vi "ASCENSOR.vi"() -> ()   [LabVIEW 2019]
panel:
  in  "Bajar":bool
  in  "Subir":bool
  in  "Posicion Ascensor":dbl(slide) scale=0.0..100.0
  in  "Selecc. Piso Inicio":enum16{"Piso 1", "Piso 2", "Piso 3", "Piso 4"}(ring)
  in  "Manual-Automatico":bool=TRUE
  in  "Start-Stop":bool
  in  "Cerrar":bool
  in  "Abrir":bool
  out "Bajando":bool
  out "Subiendo":bool
  in  "Piso 4":u16(ring)
  in  "Piso 3":u16(ring)
  in  "Piso 2":u16(ring)
  in  "Piso 1":u16(ring)
  in  "Indicador Cabina":u16(ring)
  out "Bajar 4":bool
  out "Subir 3":bool
  out "Bajar 3":bool
  out "Subir 2":bool
  out "Bajar 2":bool
  out "Subir 1":bool
  out "P02":bool
  out "P04":bool
  out "P01":bool
  out "P03":bool
  in  "Piso 4":bool
  in  "Piso 2":bool
  in  "Piso 3":bool
  in  "Piso 1":bool
  # "0 = Piso 1"
  # "33 = Piso 2"
  # "66 = Piso 3"
  # "100 = Piso 4"
  # "Operacion Manual"
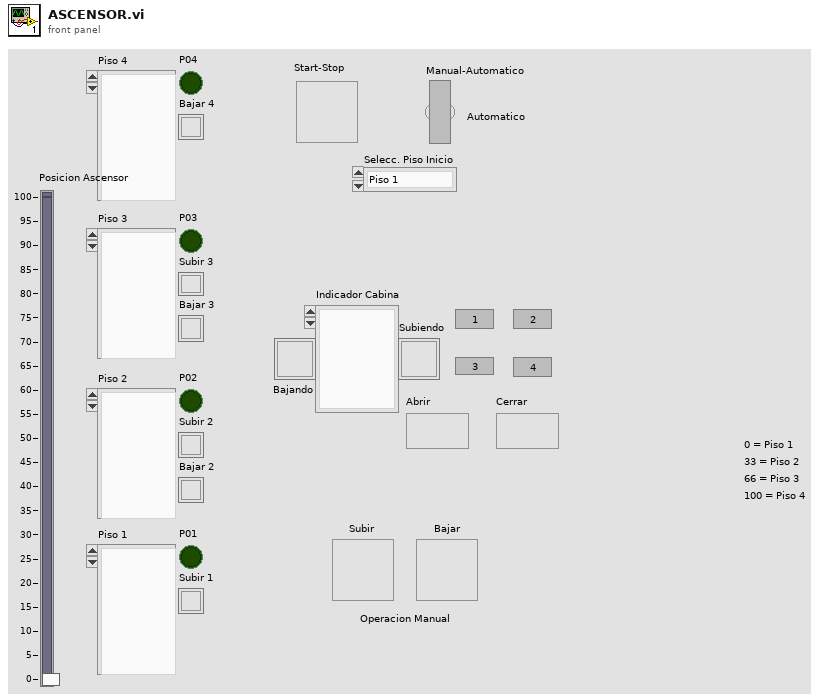
[diagram p1: front panel]
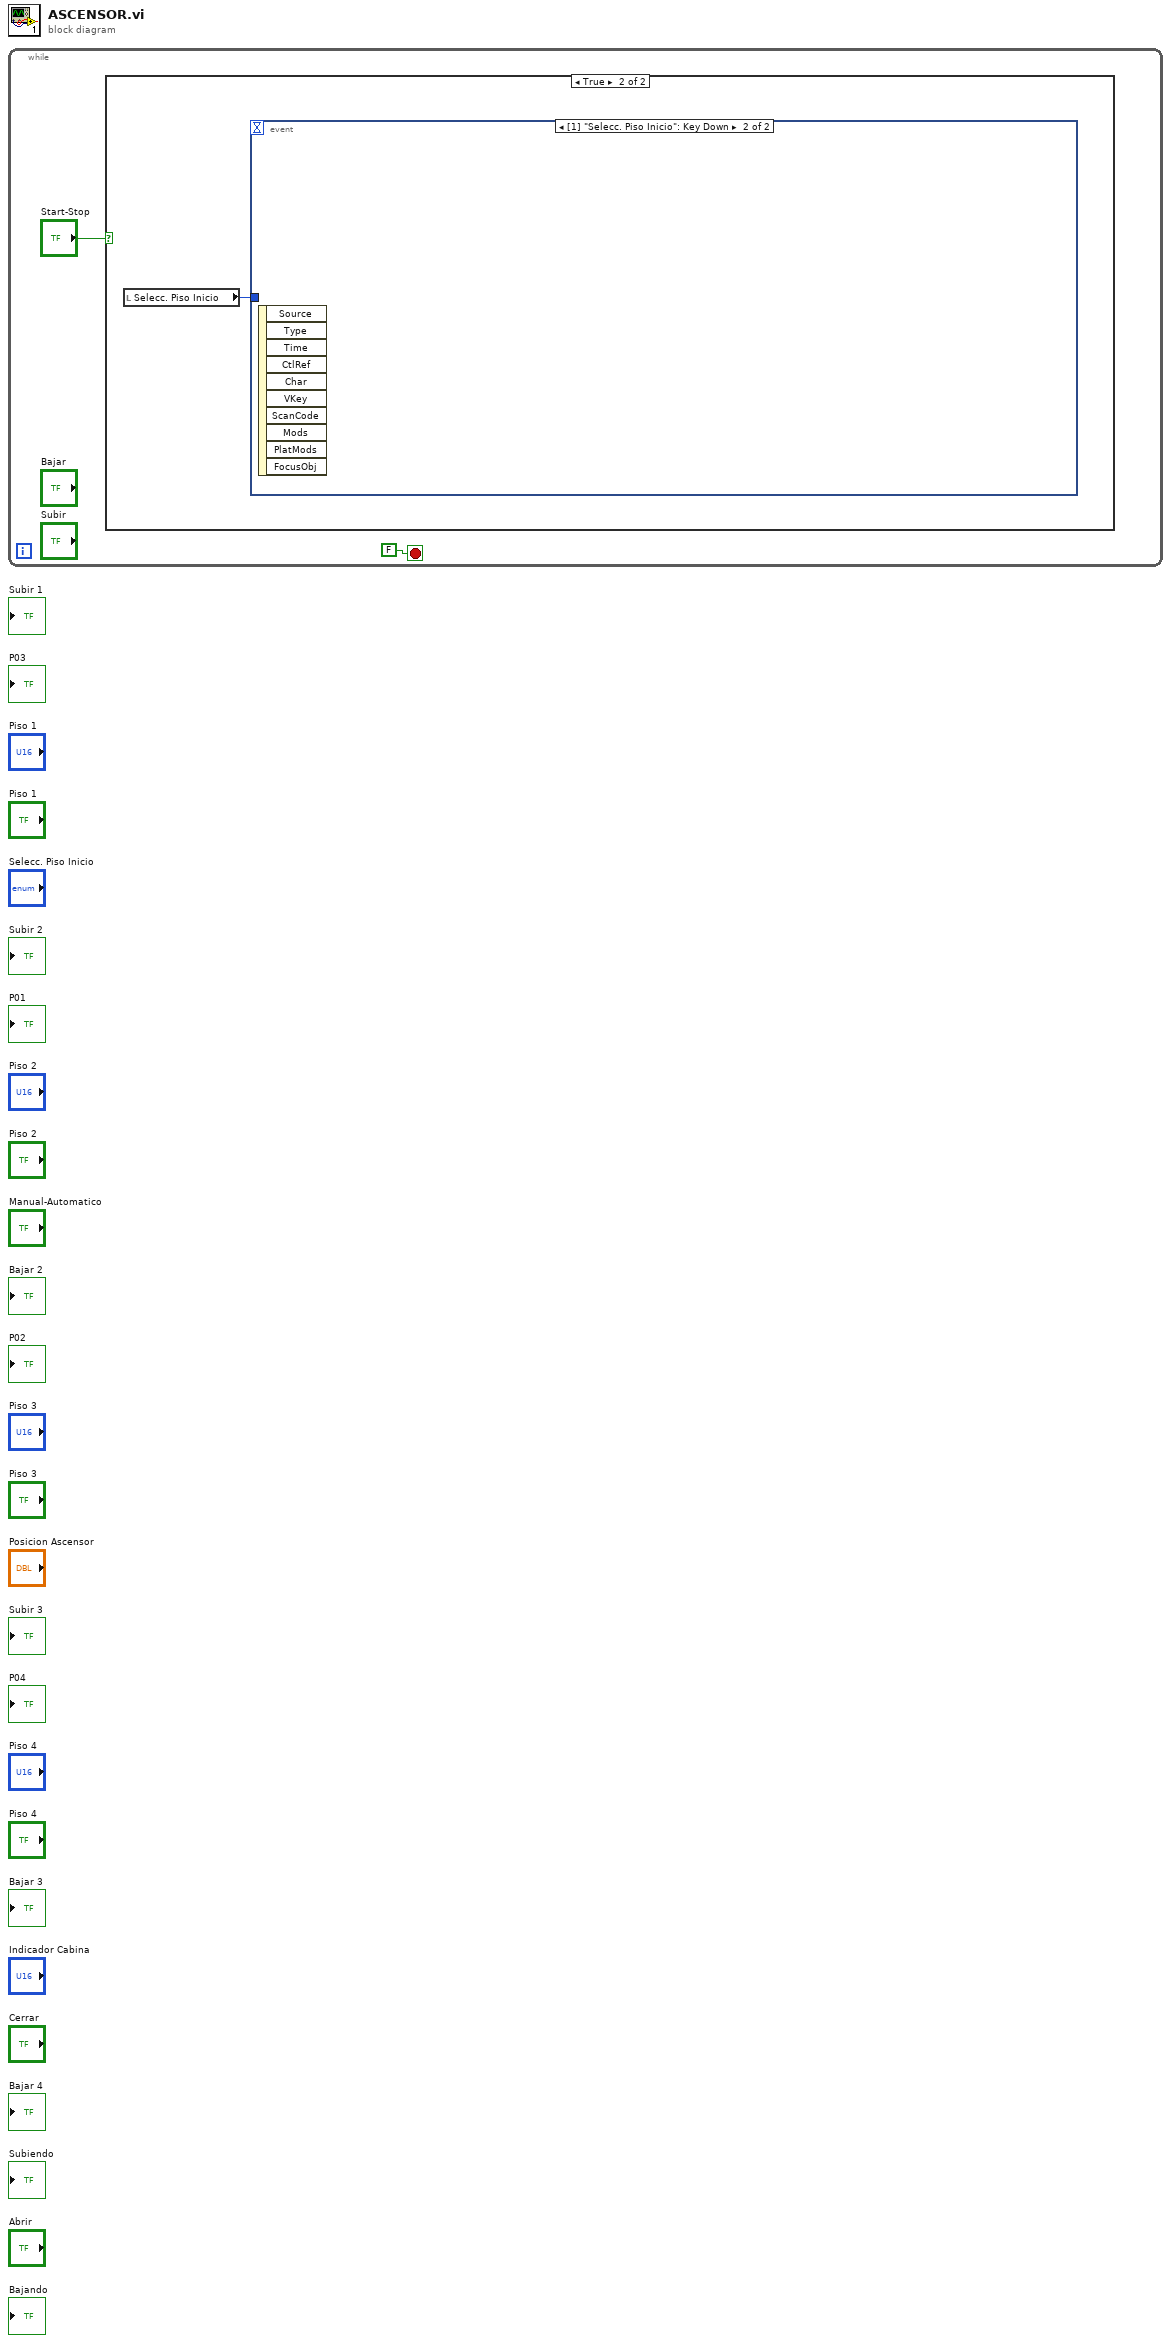
[diagram p0: block diagram]
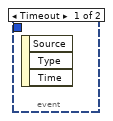
[diagram p3: hidden frame]
diagram:
  n1 = while {
    stop <- FALSE stop-if-true
    n2 = case shown="True" "Start-Stop" {
      frame False {
      }
      frame True {
        n3 = local read "Selecc. Piso Inicio"() -> (w3:enum16{"Piso 1", "Piso 2", "Piso 3", "Piso 4"})
        n4 = event shown="[1] \"Selecc. Piso Inicio\": Key Down" {
          selector: _ -> [_ _]
          dyn-events: _ -> [_ _]
          timeout: _ -> [_ _]
          tunnel: w3 -> [_ _]
          event Timeout {
            n5 = event-data() -> ()  [unwired: 1 in, 3 out]
          }
          event "Selecc. Piso Inicio": Key Down {
            n6 = event-data() -> ()  [unwired: 1 in, 10 out]
          }
        }
      }
    }
  }
